vi "LoadSBconfigParams.vi"(8 "error in (no error)":errorcluster) -> (0 "error out":errorcluster, 2 "nbar":dbl, 3 "eta":dbl)   [LabVIEW 2019]
uses:
  <vilib>/Utility/config.llb/Read Key (Double).vi
  <vilib>/Utility/config.llb/NI_LVConfig.lvlib
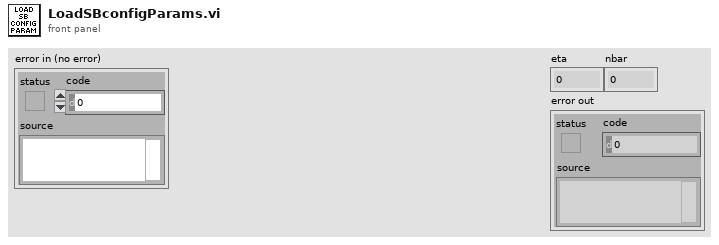
[diagram p1: front panel]
types:
  T1 = typedef "NI_LVConfig.lvlib/Config Data RefNum.ctl" = refnum<k1>
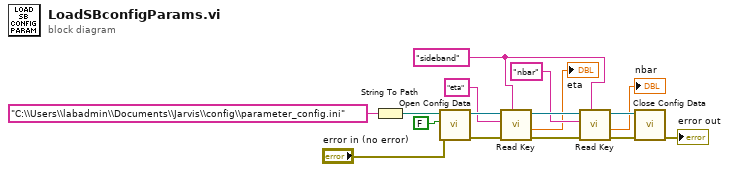
[diagram p0: block diagram]
diagram:
  w9 = "sideband" ("section")
  n1 = String To Path(string="C:\\Users\\labadmin\\Documents\\Jarvis\\config\\parameter_config.ini") -> (path=w14:path)
  n2 = call <vilib>:"Open Config Data.vi"("error in (no error)"="error in (no error)", "create file if necessary (T)"=FALSE, "configuration file path"=w14) -> ("error out"=w11:errorcluster, "refnum"=w13:T1)  [unwired: 6 in, 1 out]
  n3 = call-poly <vilib>:"Read Key.vi"("section"=w9, "error in (no error)"=w11, "key"="eta", "refnum"=w13) -> ("error out"=w10:errorcluster, "value"=→"eta":dbl, "refnum out"=w12:T1)  [unwired: 4 in, 1 out]
  n4 = call-poly <vilib>:"Read Key.vi"("section"=w9, "error in (no error)"=w10, "key"="nbar", "refnum"=w12) -> ("error out"=w5:errorcluster, "value"=→"nbar":dbl, "refnum out"=w6:T1)  [unwired: 4 in, 1 out]
  n5 = call <vilib>:"Close Config Data.vi"("error in (no error)"=w5, "refnum"=w6) -> ("error out"=→"error out":errorcluster)  [unwired: 8 in, 1 out]
